vi "PublishRequest.vi"(8 "error in (no error)":errorcluster, 9 "state":string, 10 "message":T1, 11 "service in":refnum<class "IcmMessageService.lvclass">) -> (0 "error out":errorcluster, 3 "service out":refnum<class "IcmMessageService.lvclass">)   [LabVIEW 2017, in "IcmMessageService.lvclass"]
doc: "Publishes a request to send a message to the message bus."
uses:
  <vilib>/addons/InsightCM/MessageBus/MessageService/IcmMessageService.lvclass
  <vilib>/addons/InsightCM/MessageBus/Base/controls/Message.ctl
  <vilib>/addons/InsightCM/MessageBus/Base/controls/MessageHeader.ctl
  <vilib>/addons/InsightCM/MessageBus/Base/controls/KeyValuePair.ctl
  <vilib>/addons/InsightCM/MessageBus/MessageService/IcmMessageService.lvclass/IcmMessageService.ctl
  C:/Program Files (x86)/National Instruments/LabVIEW 2017/vi.lib/addons/InsightCM/Binaries/LabviewMessageAdapter.dll
  Binaries/LabviewMessageAdapter.dll
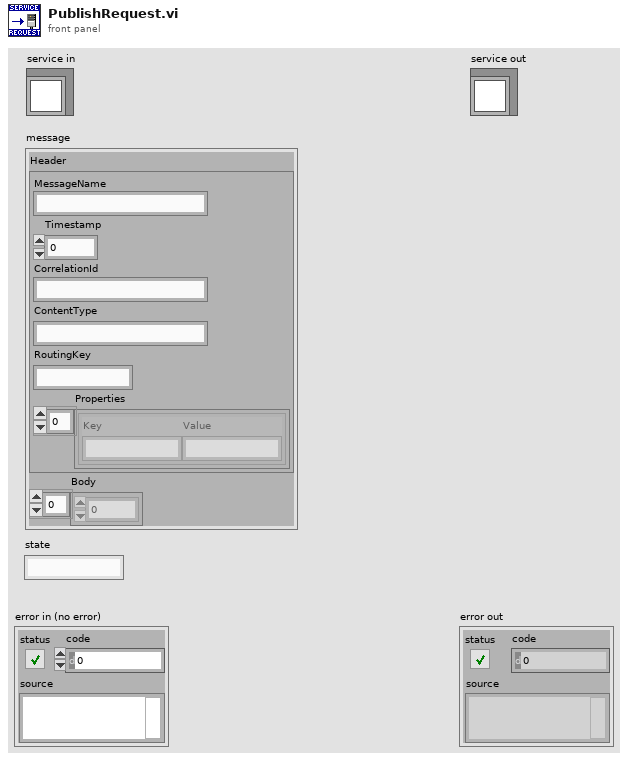
[diagram p1: front panel]
types:
  T1 = typedef "Message.ctl" = cluster{"Header":T2, "Body":u8[]}
  T2 = typedef "MessageHeader.ctl" = cluster{"MessageName":string, "Timestamp":i64, "CorrelationId":string, "ContentType":string, "RoutingKey":string, "Properties":T3[]}
  T3 = typedef "KeyValuePair.ctl" = cluster{"Key":string, "Value":string}
  T4 = typedef "MessageServiceDvr.ctl" = refnum<data-value>
  T5 = typedef "MessageServiceData.ctl" = cluster{"Service":refnum<k24>}
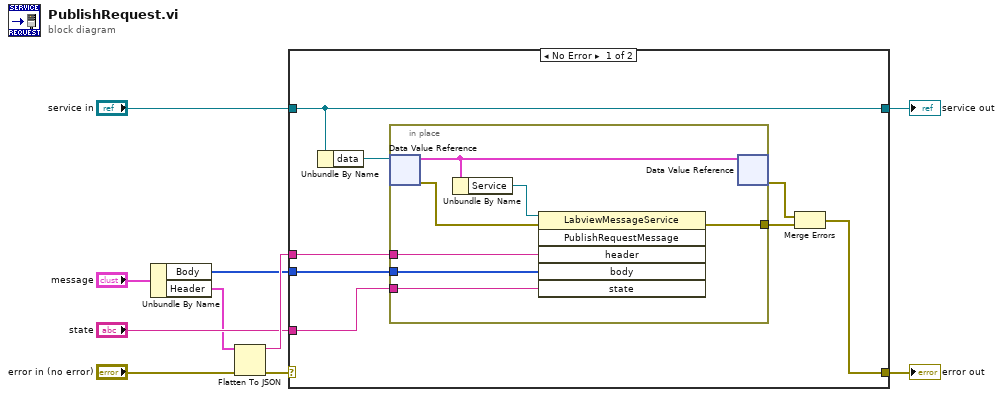
[diagram p0: block diagram]
diagram:
  n1 = Unbundle By Name("message") -> ("Body"=w1:u8[], "Header"=w2:T2)
  n2 = Flatten To JSON(anything=w2, error in (no error)="error in (no error)") -> (JSON string=w5:string, 11:w6:errorcluster)  [unwired: 1 in]
  n3 = case shown="No Error" w6 {
    selector: w6 -> [_ w27]
    tunnel: [w14 w27] -> w10
    tunnel: [w18 w26] -> w8
    tunnel: "service in" -> [w18 w26]
    tunnel: w5 -> [w13 _]
    tunnel: w1 -> [w12 _]
    tunnel: "state" -> [w11 _]
    frame No Error {
      n4 = Unbundle By Name(w18) -> ("data"=w17:T4)
      n5 = in-place {
        in-place-border: [w22] -> w15
        in-place-border: w13 -> [w21]
        in-place-border: w12 -> [w20]
        in-place-border: w11 -> [w19]
        n6 = in-place-dvr #1(w17) -> (w25:T5, w23:errorcluster)
        n7 = Unbundle By Name(w25) -> ("Service"=w24:refnum<k24>)
        n8 = invoke class="LabviewMessageService" method="PublishRequestMessage"(reference=w24, error in=w23, "header"=w21, "body"=w20, "state"=w19) -> (error out=w22:errorcluster)  [unwired: 1 in, 5 out]
        n9 = in-place-dvr #1(w25) -> (w16:errorcluster)  [unwired: 1 out]
      }
      n10 = Merge Errors(w16, w15) -> (w14:errorcluster)
    }
    frame Error {
    }
  }
  "error out" <- w10
  "service out" <- w8
